vi "NN.vi"() -> ()   [LabVIEW 2014]
panel:
  in  "Array 2":dbl[](array[numeric])
  in  "#layers":i32
  in  "Array":dbl[](array[numeric])
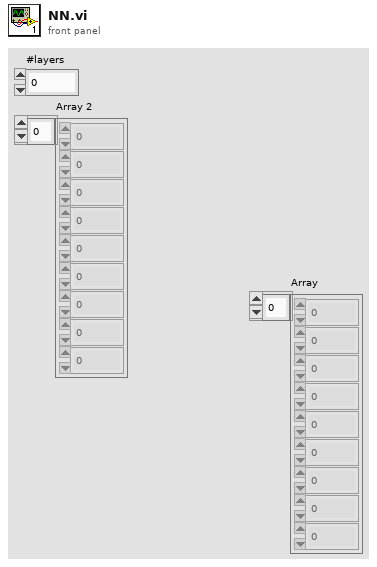
[diagram p1: front panel]
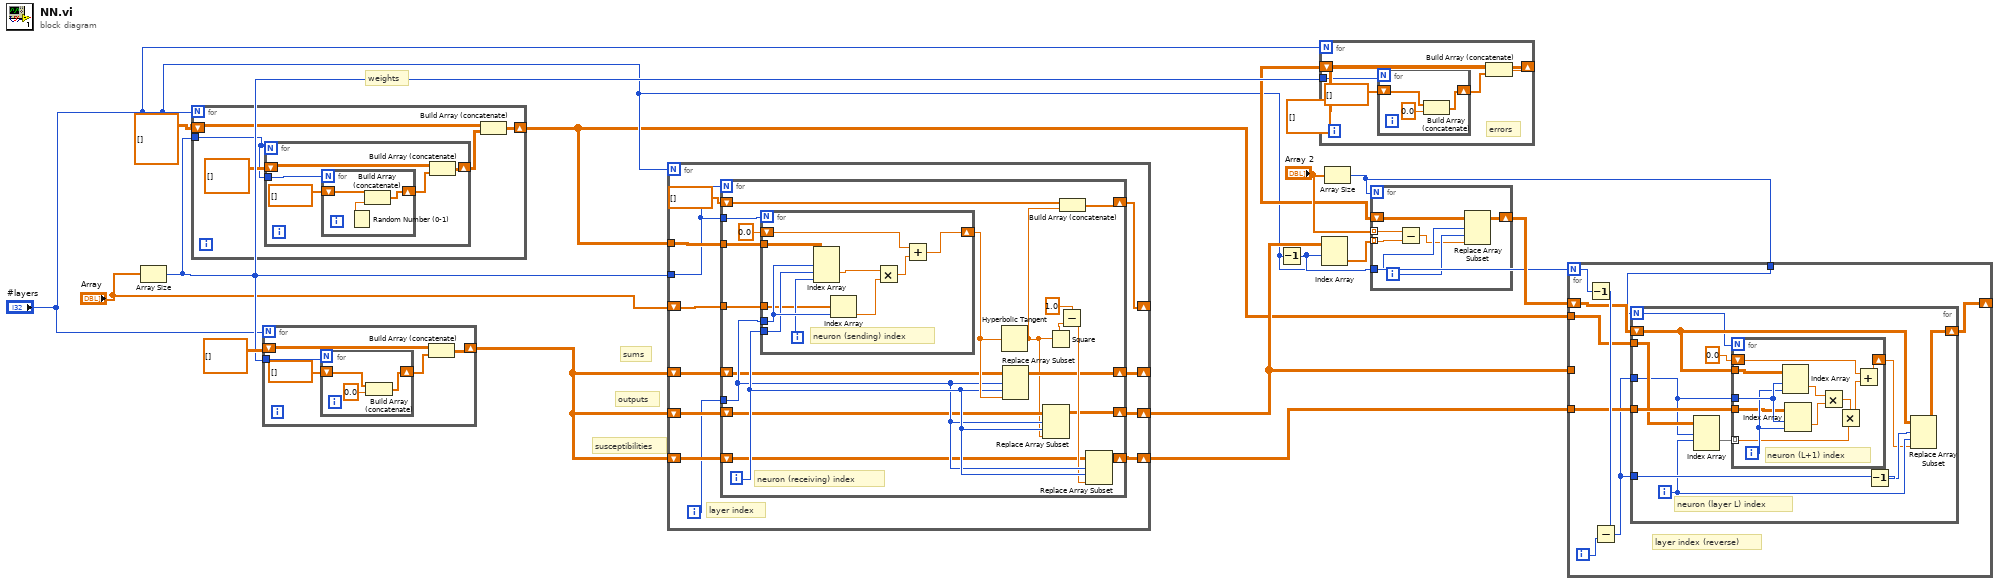
[diagram p0: block diagram]
diagram:
  # "susceptibilities"
  # "sums"
  # "outputs"
  # "weights"
  n1 = Array Size(array="Array") -> (size(s)=w13:i32)
  n2 = for {
    N: "#layers" -> [_]
    shift-right: [w20] -> w3
    shift-left: dbl[][][] [] -> [w18]
    tunnel: w13 -> [w17]
    n3 = for {
      N: w17 -> [_]
      tunnel: w17 -> [w25]
      shift-right: [w23] -> w19
      shift-left: dbl[][] [] -> [w24]
      n4 = for {
        N: w25 -> [_]
        shift-right: [w28] -> w22
        shift-left: dbl[] [] -> [w29]
        n5 = Random Number (0-1)() -> (number: 0 to 1=w27:dbl)
        n6 = Build Array (concatenate)(w29, w27) -> (w28:dbl[])
      }
      n7 = Build Array (concatenate)(w24, w22) -> (w23:dbl[][])
    }
    n8 = Build Array (concatenate)(w18, w19) -> (w20:dbl[][][])
  }
  n9 = for {
    N: "#layers" -> [_]
    shift-right: [w33] -> w1
    shift-left: dbl[][] [] -> [w34]
    tunnel: w13 -> [w31]
    n10 = for {
      N: w31 -> [_]
      shift-right: [w36] -> w32
      shift-left: dbl[] [] -> [w35]
      n11 = Build Array (concatenate)(w35, 0.0 ("element")) -> (w36:dbl[])
    }
    n12 = Build Array (concatenate)(w34, w32) -> (w33:dbl[][])
  }
  n13 = for {
    N: "#layers" -> [_]
    tunnel: w3 -> [w49]
    tunnel: w13 -> [w41]
    shift-right: [w38] -> _
    shift-left: "Array" -> [w39]
    shift-right: [w44] -> w8
    shift-left: w1 -> [w48]
    shift-right: [w43] -> w9
    shift-left: w1 -> [w47]
    shift-right: [w45] -> _
    shift-left: w1 -> [w46]
    i -> [w42]
    # "layer index"
    n14 = for {
      N: w41 -> [_]
      tunnel: w49 -> [w68]
      tunnel: w42 -> [w62]
      shift-right: [w57] -> w44
      shift-left: w48 -> [w58]
      shift-right: [w56] -> w43
      shift-left: w47 -> [w59]
      shift-right: [w55] -> w45
      shift-left: w46 -> [w60]
      tunnel: w41 -> [w54]
      shift-right: [w52] -> w38
      shift-left: dbl[] [] -> [w51]
      tunnel: w39 -> [w50]
      i -> [w63]
      # "neuron (receiving) index"
      n15 = for {
        N: w54 -> [_]
        tunnel: w68 -> [w78]
        tunnel: w63 -> [w71]
        tunnel: w62 -> [w77]
        shift-right: [w73] -> w66
        shift-left: 0.0 -> [w74]
        tunnel: w50 -> [w70]
        i -> [w72]
        # "neuron (sending) index"
        n16 = Index Array(array=w78, index (dim 0)=w77, index (dim 1)=w71, index (dim 2)=w72) -> (element=w76:dbl)
        n17 = Index Array(array=w70, index=w77) -> (element=w69:dbl)
        n18 = Multiply(x=w76, y=w69) -> (x*y=w75:dbl)
        n19 = Add(x=w74, y=w75) -> (x+y=w73:dbl)
      }
      n20 = Hyperbolic Tangent(1:w66) -> (0:w53:dbl)
      n21 = Replace Array Subset(array=w60, new element=w66, index (row)=w62, index (col)=w63) -> (w55:dbl[][])
      n22 = Replace Array Subset(array=w59, new element=w53, index (row)=w62, index (col)=w63) -> (w56:dbl[][])
      n23 = Square(x=w53) -> (x^2=w64:dbl)
      n24 = Subtract(x=1.0, y=w64) -> (x-y=w61:dbl)
      n25 = Build Array (concatenate)(w51, w53) -> (w52:dbl[])
      n26 = Replace Array Subset(array=w58, new element=w61, index (row)=w62, index (col)=w63) -> (w57:dbl[][])
    }
  }
  n27 = Decrement(x="#layers") -> (x-1=w6:i32)
  n28 = for {
    N: "#layers" -> [_]
    shift-right: [w81] -> w7
    shift-left: dbl[][] [] -> [w82]
    tunnel: w13 -> [w79]
    # "errors"
    n29 = for {
      N: w79 -> [_]
      shift-right: [w85] -> w80
      shift-left: dbl[] [] -> [w84]
      n30 = Build Array (concatenate)(w84, 0.0 ("element")) -> (w85:dbl[])
    }
    n31 = Build Array (concatenate)(w82, w80) -> (w81:dbl[][])
  }
  n32 = Index Array(array=w9, index (row)=w6) -> (element=w10:dbl[])  [unwired: 1 in]
  n33 = Array Size(array="Array 2") -> (size(s)=w2:i32)
  n34 = for {
    N: w2 -> [_]
    tunnel: "Array 2" -> [w93] mode=indexing
    tunnel: w10 -> [w92] mode=indexing
    shift-right: [w87] -> w5
    shift-left: w7 -> [w91]
    tunnel: w6 -> [w90]
    i -> [w89]
    n35 = Subtract(x=w93, y=w92) -> (x-y=w88:dbl)
    n36 = Replace Array Subset(array=w91, new element=w88, index (row)=w90, index (col)=w89) -> (w87:dbl[][])
  }
  n37 = for {
    N: "#layers" -> [w101]
    tunnel: w9 -> [_]
    tunnel: w8 -> [w98]
    shift-right: [w94] -> _
    shift-left: w5 -> [w99]
    tunnel: w3 -> [w97]
    tunnel: w2 -> [w95]
    i -> [w102]
    # "layer index (reverse)"
    n38 = Decrement(x=w101) -> (x-1=w100:i32)
    n39 = Subtract(x=w100, y=w102) -> (x-y=w96:i32)
    n40 = for {
      N: w95 -> [w104]
      tunnel: w96 -> [w112]
      tunnel: w98 -> [w114]
      tunnel: w97 -> [w113]
      tunnel: w96 -> [w109]
      shift-right: [w103] -> w94
      shift-left: w99 -> [w110]
      i -> [w107]
      # "neuron (layer L) index"
      n41 = Index Array(array=w113, index (dim 0)=w112, index (dim 1)=w107) -> (element=w111:dbl[])  [unwired: 1 in]
      n42 = for {
        N: w104 -> [_]
        tunnel: w110 -> [w125]
        shift-right: [w122] -> w106
        shift-left: 0.0 -> [w123]
        tunnel: w112 -> [w121]
        tunnel: w114 -> [w115]
        tunnel: w111 -> [w117] mode=indexing
        i -> [w120]
        # "neuron (L+1) index"
        n43 = Index Array(array=w125, index (row)=w121, index (col)=w120) -> (element=w124:dbl)
        n44 = Index Array(array=w115, index (row)=w121, index (col)=w120) -> (element=w119:dbl)
        n45 = Multiply(x=w124, y=w119) -> (x*y=w118:dbl)
        n46 = Multiply(x=w118, y=w117) -> (x*y=w116:dbl)
        n47 = Add(x=w123, y=w116) -> (x+y=w122:dbl)
      }
      n48 = Decrement(x=w109) -> (x-1=w108:i32)
      n49 = Replace Array Subset(array=w110, new element=w106, index (row)=w108, index (col)=w107) -> (w103:dbl[][])
    }
  }
